vi "Graphs.vi"() -> ()   [LabVIEW 2017]
panel:
  out "Output Chart":T1(graph)={"OutputCount"=4, "Numeric Control"=0}
  out "Time Chart":T2(graph)={"Index"=0.0, "TF"=10.004, "Insert"=0.785, "Cutting"=0.897, "PF"=8.0, "Measure."=0.484, "Reject"=0.813}
  out "OEE Chart":T3(graph)={"AVL"=84.48712976789105, "PRF"=46.043358451551796, "QUA"=91.75257731958763, "OEE"=35.69240585976024}
  out "Measurement Chart":T4(graph)={"1"=189.43338537216187, "2"=188.73366138458252, "3"=189.30836337280275, "4"=188.44248421859743, "4"=187.9, "4"=189.9}
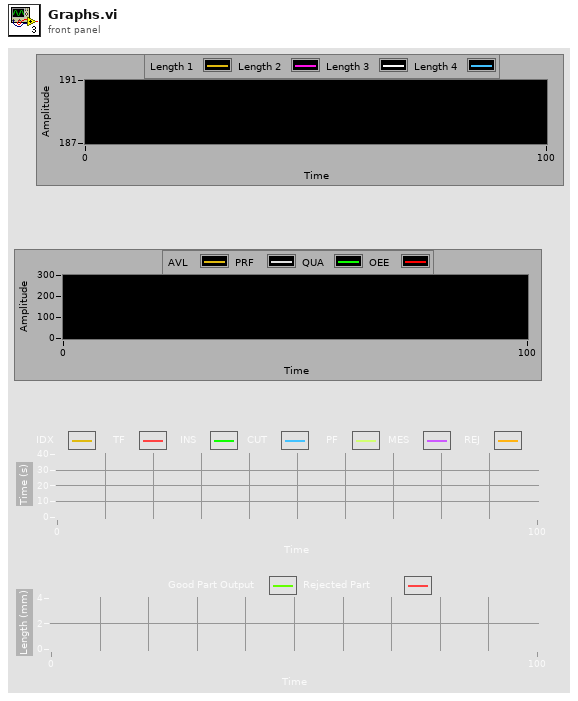
[diagram p1: front panel]
types:
  T1 = cluster{"OutputCount":u32, "Numeric Control":u32}
  T2 = cluster{"Index":dbl, "TF":dbl, "Insert":dbl, "Cutting":dbl, "PF":dbl, "Measure.":dbl, "Reject":dbl}
  T3 = cluster{"AVL":dbl, "PRF":dbl, "QUA":dbl, "OEE":dbl}
  T4 = cluster{"1":dbl, "2":dbl, "3":dbl, "4":dbl, "4":dbl, "4":dbl}
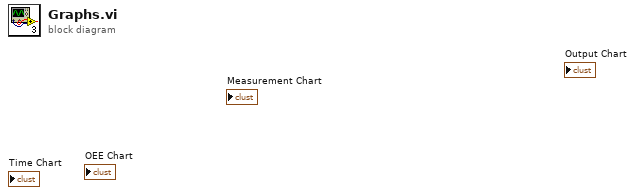
[diagram p0: block diagram]
diagram:
